vi "Configure Math.vi"(0 "VISA resource name":refnum<visa-resource-name>, 1 "Operation (0:None)":T1(ring), 2 "Internal Storage (T: Enabled)":bool=TRUE, 5 "Null Offset (0.00)":dbl format="%_3f", 7 "dB Reference Point (0.00 dB)":dbl format="%.2f", 9 "dBm Impedance (600 Ohms)":i32(ring)=600 items=["50"=50, "75"=75, "93"=93, "110"=110, "124"=124, "125"=125, "135"=135, "150"=150, "250"=250, "300"=300, "500"=500, "600"=600, "800"=800, "900"=900, "1000"=1000, "1200"=1200, "8000"=8000], 11 "error in (no error)":errorcluster, 12 "Upper Limit (0.00)":dbl format="%.2f", 13 "Lower Limit (0.00)":dbl format="%.2f") -> (4 "VISA resource name out":refnum<visa-resource-name>, 15 "error out":errorcluster)   [LabVIEW 2014, in "Fluke 884X Series.lvlib"]
doc: "Configures the math functions available on the instrument."
uses:
  Fluke 884X Series.lvlib
panel:
  # "Limit"
  # "DB Measurements"
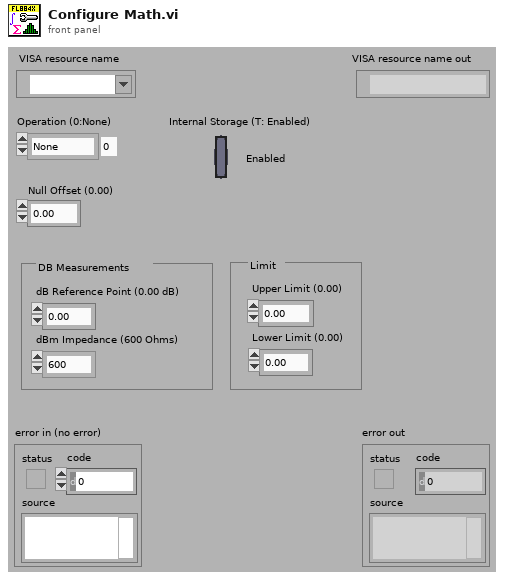
[diagram p1: front panel]
types:
  T1 = enum16{"None", "Min/Max", "Null", "dB", "dBm", "Limit"}
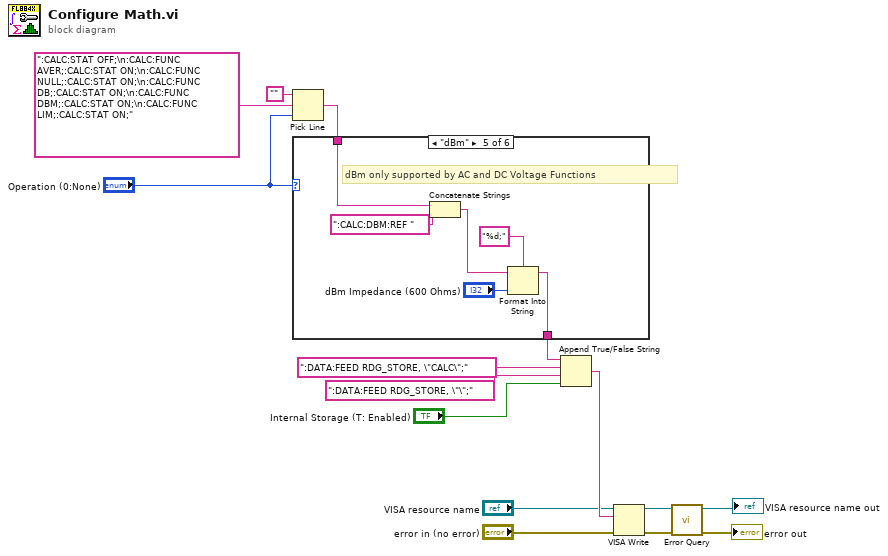
[diagram p0: block diagram]
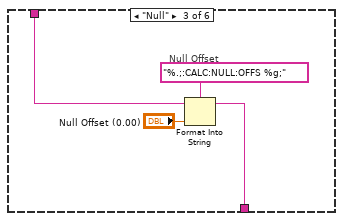
[diagram p4: hidden frame]
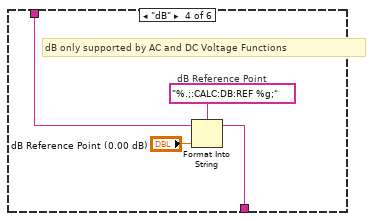
[diagram p5: hidden frame]
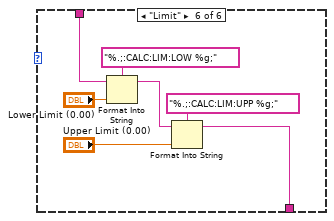
[diagram p6: hidden frame]
diagram:
  # "Math Function"
  n1 = Pick Line(string ("")="" ("Empty String Constant"), multi-line string=":CALC:STAT OFF;\n:CALC:FUNC AVER;:CALC:STAT ON;\n:CALC:FUNC NULL;:CALC:STAT ON;\n:CALC:FUNC DB;:CALC:STAT ON;\n:CALC:FUNC DBM;:CALC:STAT ON;\n:CALC:FUNC LIM;:CALC:STAT ON;", line index="Operation (0:None)") -> (output string=w14:string)
  n2 = case shown="\"dBm\"" "Operation (0:None)" {
    tunnel: w14 -> [w16 w17 w21 w25 w31 w38]
    tunnel: [w16 w17 w20 w23 w26 w32] -> w6
    frame "None", Default {
    }
    frame "Min/Max" {
    }
    frame "Null" {
      # "Null Offset"
      n3 = Format Into String(format string="%.;:CALC:NULL:OFFS %g;", initial string=w21, "Null Offset (0.00)") -> (resulting string=w20:string)  [unwired: 1 in, 1 out]
    }
    frame "dB" {
      # "dB only supported by AC and DC Voltage Functions"
      # "dB Reference Point"
      n4 = Format Into String(format string="%.;:CALC:DB:REF %g;", initial string=w25, "dB Reference Point (0.00 dB)") -> (resulting string=w23:string)  [unwired: 1 in, 1 out]
    }
    frame "dBm" {
      # "dBm only supported by AC and DC Voltage Functions"
      n5 = Concatenate Strings(w31, ":CALC:DBM:REF ") -> (w29:string)
      n6 = Format Into String(format string="%d;", initial string=w29, "dBm Impedance (600 Ohms)") -> (resulting string=w26:string)  [unwired: 1 in, 1 out]
    }
    frame "Limit" {
      n7 = Format Into String(format string="%.;:CALC:LIM:LOW %g;", initial string=w38, "Lower Limit (0.00)") -> (resulting string=w33:string)  [unwired: 1 in, 1 out]
      n8 = Format Into String(format string="%.;:CALC:LIM:UPP %g;", initial string=w33, "Upper Limit (0.00)") -> (resulting string=w32:string)  [unwired: 1 in, 1 out]
    }
  }
  n9 = Append True/False String(1:"Internal Storage (T: Enabled)", 2:":DATA:FEED RDG_STORE, \"\";" ("true string"), 3:":DATA:FEED RDG_STORE, \"CALC\";" ("true string"), 4:w6) -> (0:w5:string)
  n10 = VISA Write(VISA resource name="VISA resource name", write buffer=w5, error in (no error)="error in (no error)") -> (VISA resource name out=w11:refnum<visa-resource-name>, error out=w12:errorcluster)  [unwired: 1 out]
  n11 = call "Error Query.vi"("error in (no error)"=w12, "VISA resource name"=w11) -> ("error out"=→"error out":errorcluster, "VISA resource name out"=→"VISA resource name out":refnum<visa-resource-name>)  [unwired: 6 in, 2 out]
